vi "SignalInfo.vi"(6 "Error in":errorcluster, 8 "Signal":refnum<k24>, 9 "DevicesAndSignals":T2) -> (0 "Error out":errorcluster, 2 "SignalInfo":T1, 3 "DevicesAndSignals":T2)   [LabVIEW 2016]
doc: "Delivers various signal properties.\n\nSignal: Signal whose properties should be read\nSignalInfo: Cluster that contains information about the signal"
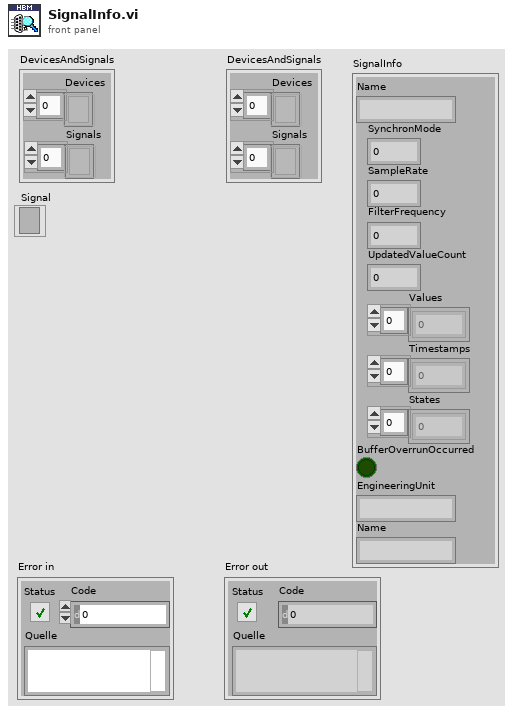
[diagram p1: front panel]
types:
  T1 = cluster{"Name":string, "SynchronMode":i32, "SampleRate":dbl, "FilterFrequency":dbl, "UpdatedValueCount":i32, "Values":dbl[], "Timestamps":dbl[], "States":i32[], "BufferOverrunOccurred":bool, "EngineeringUnit":string, "Name":string}
  T2 = cluster{"Devices":refnum<k24>[], "Signals":refnum<k24>[]}
  T3 = cluster{"Name":string, "SynchronMode":i32, "SampleRate":dbl, "Frequency":dbl, "UpdatedValueCount":i32, "Values":dbl[], "Timestamps":dbl[], "States":i32[], "BufferOverrunOccurred":bool, "EngineeringUnit":string, "Name":string}
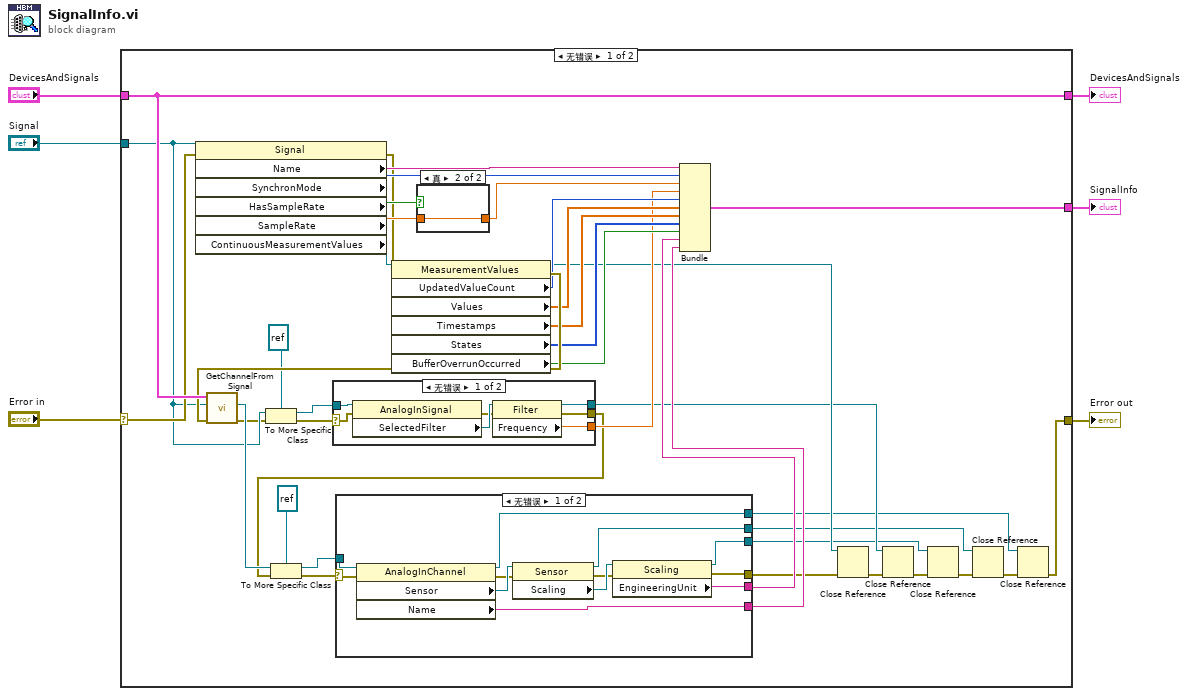
[diagram p0: block diagram]
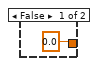
[diagram p4: hidden frame]
diagram:
  n1 = case shown="无错误" "Error in" {
    selector: "Error in" -> [w38 w69]
    tunnel: [w13 w69] -> w6
    tunnel: "Signal" -> [w32 _]
    tunnel: [w33 _] -> w1
    tunnel: "DevicesAndSignals" -> [w39 w68]
    tunnel: [w39 w68] -> w2
    frame No Error {
      n2 = property on="Eigenschaftsknoten" class="Signal"(reference=w32, error in=w38) -> (error out=w40:errorcluster, "Name"=w45:string, "SynchronMode"=w44:i32, "HasSampleRate"=w43:bool, "SampleRate"=w42:dbl, "ContinuousMeasurementValues"=w46:refnum<k24>)  [unwired: 1 out]
      n3 = property on="Eigenschaftsknoten" class="MeasurementValues"(reference=w46, error in=w40) -> (reference out=w16:refnum<k24>, error out=w37:errorcluster, "UpdatedValueCount"=w23:i32, "Values"=w24:dbl[], "Timestamps"=w25:dbl[], "States"=w26:i32[], "BufferOverrunOccurred"=w27:bool)
      n4 = call "GetChannelFromSignal.vi"("Error in"=w37, "Signal"=w32, "DevicesAndSignals"=w39) -> ("Error out"=w19:errorcluster, "Channel"=w36:refnum<k24>)  [unwired: 6 in, 1 out]
      n5 = To More Specific Class(target class=refnum<k24> refnum (".NET (Referenz)"), reference=w32, error in=w19) -> (specific class reference=w30:refnum<k24>, error out=w31:errorcluster)
      n6 = case shown="无错误" w31 {
        selector: w31 -> [w50 _]
        tunnel: w30 -> [w53 _]
        tunnel: [w51 _] -> w22
        tunnel: [w48 _] -> w18
        tunnel: [w47 _] -> w10
        frame No Error {
          n7 = property on="Eigenschaftsknoten" class="AnalogInSignal"(reference=w53, error in=w50) -> (error out=w49:errorcluster, "SelectedFilter"=w52:refnum<k24>)  [unwired: 1 out]
          n8 = property on="Eigenschaftsknoten" class="Filter"(reference=w52, error in=w49) -> (reference out=w47:refnum<k24>, error out=w48:errorcluster, "Frequency"=w51:dbl)
        }
        frame Error {
        }
      }
      n9 = To More Specific Class(target class=refnum<k24> refnum (".NET (Referenz)"), reference=w36, error in=w18) -> (specific class reference=w35:refnum<k24>, error out=w34:errorcluster)
      n10 = case shown="无错误" w34 {
        selector: w34 -> [w60 _]
        tunnel: w35 -> [w65 _]
        tunnel: [w59 _] -> w28
        tunnel: [w58 _] -> w29
        tunnel: [w57 _] -> w17
        tunnel: [w56 _] -> w7
        tunnel: [w55 _] -> w8
        tunnel: [w54 _] -> w9
        frame No Error {
          n11 = property on="Eigenschaftsknoten" class="AnalogInChannel"(reference=w65, error in=w60) -> (reference out=w56:refnum<k24>, error out=w62:errorcluster, "Sensor"=w63:refnum<k24>, "Name"=w58:string)
          n12 = property on="Eigenschaftsknoten" class="Sensor"(reference=w63, error in=w62) -> (reference out=w55:refnum<k24>, error out=w61:errorcluster, "Scaling"=w64:refnum<k24>)
          n13 = property on="Eigenschaftsknoten" class="Scaling"(reference=w64, error in=w61) -> (reference out=w54:refnum<k24>, error out=w57:errorcluster, "EngineeringUnit"=w59:string)
        }
        frame Error {
        }
      }
      n14 = case shown="真" w43 {
        tunnel: w42 -> [_ w67]
        tunnel: [0.0 ("SampleRate") w67] -> w41
        frame False {
        }
        frame True {
        }
      }
      n15 = Bundle("Name"=w45, "SynchronMode"=w44, "SampleRate"=w41, "Frequency"=w22, "UpdatedValueCount"=w23, "Values"=w24, "Timestamps"=w25, "States"=w26, "BufferOverrunOccurred"=w27, "EngineeringUnit"=w28, "Name"=w29) -> (w33:T3)  [unwired: 1 in]
      n16 = Close Reference(reference=w16, error in (no error)=w17) -> (error out=w12:errorcluster)
      n17 = Close Reference(reference=w10, error in (no error)=w12) -> (error out=w11:errorcluster)
      n18 = Close Reference(reference=w9, error in (no error)=w11) -> (error out=w15:errorcluster)
      n19 = Close Reference(reference=w8, error in (no error)=w15) -> (error out=w14:errorcluster)
      n20 = Close Reference(reference=w7, error in (no error)=w14) -> (error out=w13:errorcluster)
    }
    frame Error {
    }
  }
  "Error out" <- w6
  "DevicesAndSignals" <- w2
  "SignalInfo" <- w1
